vi "Write Random Message.vi"(8 "error in":errorcluster, 9 "Send Message?":bool, 11 "Queue in":refnum<queue>) -> (0 "error out":errorcluster, 3 "Queue out":refnum<queue>)   [LabVIEW 2018]
uses:
  Support/Message Queue/Message Cluster.ctl
  Support/Message Queue/Enqueue Message (Single).vi
  Support/Message Queue/Message Queue.lvlib
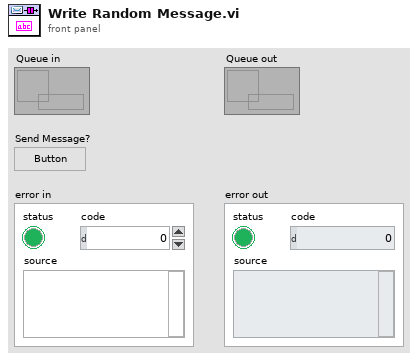
[diagram p1: front panel]
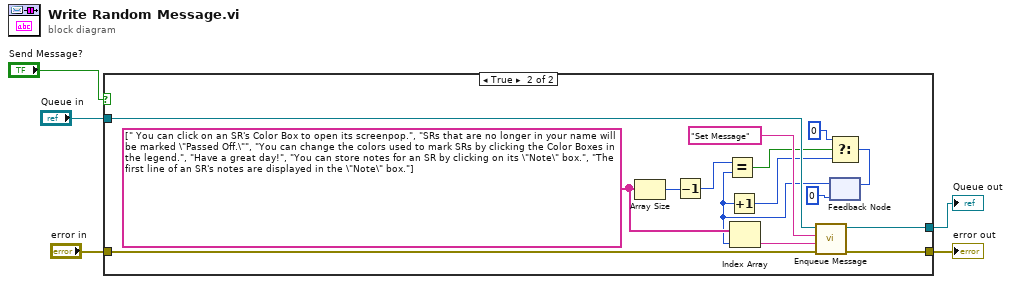
[diagram p0: block diagram]
diagram:
  n1 = case shown="True" "Send Message?" {
    tunnel: "error in" -> [w6 w22]
    tunnel: [w6 w21] -> w4
    tunnel: [w7 w19] -> w3
    tunnel: "Queue in" -> [w7 w18]
    frame False {
    }
    frame True {
      w16 = string[] [" You can click on an SR's Color Box to open its screenpop.", "SRs that are no longer in your name will be marked \"Passed Off.\"", "You can change the colors used to mark SRs by clicking the Color Boxes in the legend.", "Have a great day!", "You can store notes for an SR by clicking on its \"Note\" box.", "The first line of an SR's notes are displayed in the \"Note\" box."]
      n2 = Array Size(array=w16) -> (size(s)=w15:i32)
      n3 = Decrement(x=w15) -> (x-1=w14:i32)
      n4 = feedback #1(0 ("index")) -> (w13:i32)
      n5 = Equal?(x=w14, y=w13) -> (x = y?=w12:bool)
      n6 = Increment(x=w13) -> (x+1=w11:i32)
      n7 = Index Array(array=w16, index=w13) -> (element=w8:string)
      n8 = call-poly "Enqueue Message.vi"("error in (no error)"=w22, "Message Data"=w8, "Message"="Set Message", "Message Queue"=w18) -> ("error out"=w21:errorcluster, "dup Message Queue"=w19:refnum<queue>)  [unwired: 6 in]
      n9 = Select(t=0, s=w12, f=w11) -> (s? t:f=w9:i32)
      n10 = feedback-in #1(w9) -> ()
    }
  }
  "error out" <- w4
  "Queue out" <- w3
